vi "Array.vi"() -> (2 "Startlinie true":bool, 3 "array":bool[](array[boolean]))   [LabVIEW 2016]
doc: "VI berrechnet Abweichung des Linearray zur Mittellinie\n05.04.17_Tloe"
uses:
  <vilib>/myRIO/Instrument Drivers/Onboard IO/DIO/typedefs/DIO Reference.ctl
  <vilib>/myRIO/Common/Instrument Driver Framework/Utilities/typedefs/myRIO Generic Hardware Reference.ctl
  <vilib>/myRIO/Common/Instrument Driver Framework/Utilities/typedefs/Hardware Version Enum.ctl
  <vilib>/myRIO/Common/Instrument Driver Framework/Utilities/typedefs/myRIO v1.0 Reference.ctl
  <vilib>/myRIO/Common/Instrument Driver Framework/Utilities/typedefs/Generic FPGA Reference.ctl
  <vilib>/myRIO/Common/Instrument Driver Framework/myRIO v1.0/DIO/typedefs/DIO Channels List.ctl
  <vilib>/myRIO/Common/Instrument Driver Framework/myRIO v1.0/DIO/typedefs/DIO Channels Enum.ctl
  <vilib>/userdefined/High Color/nirio_resource_hc.ctl
  <vilib>/myRIO/Common/Instrument Driver Framework/Utilities/vis/Is FPGA Ref Available.vi
  <vilib>/myRIO/Common/Instrument Driver Framework/myRIO v1.0/DIO/vis/myRIO v1.1 Open DIO.vi
  <vilib>/myRIO/Instrument Drivers/Onboard IO/DIO/vis/Read.vi
  <vilib>/myRIO/Common/Instrument Driver Framework/Utilities/vis/Validate Channels.vi
  <vilib>/myRIO/Common/Instrument Driver Framework/myRIO v1.0/DIO/vis/myRIO v1.0 Reserve DIO.vi
  <vilib>/myRIO/Common/Instrument Driver Framework/myRIO v1.0/Resource Manager/vis/myRIO v1.0 Reserve Channel List.vi
  <vilib>/myRIO/Common/Instrument Driver Framework/myRIO v1.0/DIO/vis/myRIO v1.0 Build MUX Configuration DIO.vi
  <vilib>/myRIO/Common/Instrument Driver Framework/myRIO v1.0/Resource Manager/vis/myRIO v1.0 Reserve Channel.vi
  <vilib>/myRIO/Common/Instrument Driver Framework/myRIO v1.0/Resource Manager/vis/myRIO v1.0 Unreserve Channel.vi
  <vilib>/myRIO/Common/Instrument Driver Framework/myRIO v1.0/Resource Manager/vis/myRIO v1.0 Create Configuration List.vi
  <vilib>/myRIO/Common/Instrument Driver Framework/myRIO v1.0/Resource Manager/vis/myRIO v1.0 Build Mutex Name.vi
  <vilib>/Utility/VariantDataType/GetNumericInfo.vi
  <vilib>/Utility/error.llb/Error Cluster From Error Code.vi
  <vilib>/myRIO/Common/Instrument Driver Framework/myRIO v1.0/myRIO v1.1 Open.vi
  <vilib>/myRIO/Common/Instrument Driver Framework/Utilities/vis/IO Manager.vi
  <vilib>/myRIO/Common/Instrument Driver Framework/Utilities/vis/Configuration Manager.vi
  <vilib>/myRIO/Common/Instrument Driver Framework/myRIO v1.0/Resource Manager/vis/myRIO v1.0 Configure IO.vi
  <vilib>/myRIO/Common/Instrument Driver Framework/myRIO v1.0/myRIO v1.0 Close.vi
  <vilib>/myRIO/Common/Instrument Driver Framework/myRIO v1.0/DIO/vis/myRIO v1.0 Read DIO.vi
  <vilib>/myRIO/Express VI/Onboard IO/DI/DI Express VI.xnode
  <vilib>/myRIO/Instrument Drivers/Onboard IO/DIO/vis/myRIO DIO Open.xnode
  <vilib>/myRIO/Instrument Drivers/Onboard IO/DIO/DIO.lvlib
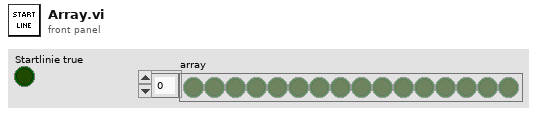
[diagram p1: front panel]
types:
  T1 = cluster{"A/DIO0 (Pin 11)":bool, "A/DIO1 (Pin 13)":bool, "A/DIO2 (Pin 15)":bool, "A/DIO3 (Pin 17)":bool, "A/DIO4 (Pin 19)":bool, "A/DIO5 (Pin 21)":bool, "A/DIO6 (Pin 23)":bool, "A/DIO7 (Pin 25)":bool, "B/DIO7 (Pin 25)":bool, "B/DIO6 (Pin 23)":bool, "B/DIO5 (Pin 21)":bool, "B/DIO3 (Pin 17)":bool, "B/DIO4 (Pin 19)":bool, "B/DIO2 (Pin 15)":bool, "B/DIO1 (Pin 13)":bool, "B/DIO12 (Pin 22)":bool}
  T2 = cluster{"A/DIO0 (Pin 11)":i16, "A/DIO1 (Pin 13)":i16, "A/DIO2 (Pin 15)":i16, "A/DIO3 (Pin 17)":i16, "A/DIO4 (Pin 19)":i16, "A/DIO5 (Pin 21)":i16, "A/DIO6 (Pin 23)":i16, "A/DIO7 (Pin 25)":i16, "B/DIO7 (Pin 25)":i16, "B/DIO6 (Pin 23)":i16, "B/DIO5 (Pin 21)":i16, "B/DIO3 (Pin 17)":i16, "B/DIO4 (Pin 19)":i16, "B/DIO2 (Pin 15)":i16, "B/DIO1 (Pin 13)":i16, "B/DIO12 (Pin 22)":i16}
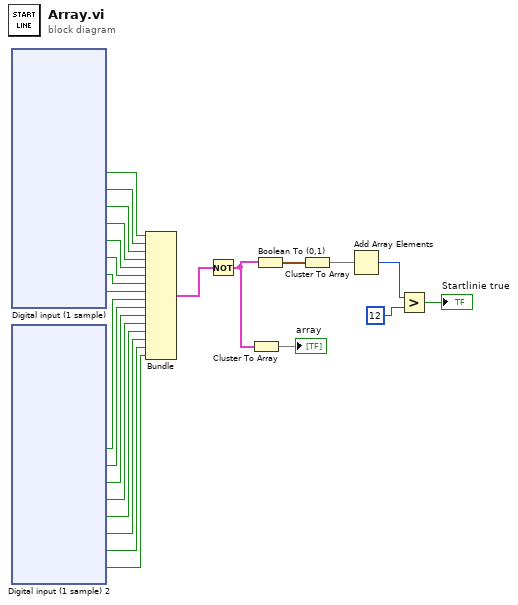
[diagram p0: block diagram]
diagram:
  n1 = xnode "Digital input (1 sample)"() -> ("A/DIO0 (Pin 11)"=w15:bool, "A/DIO1 (Pin 13)"=w16:bool, "A/DIO2 (Pin 15)"=w17:bool, "A/DIO3 (Pin 17)"=w18:bool, "A/DIO4 (Pin 19)"=w19:bool, "A/DIO5 (Pin 21)"=w20:bool, "A/DIO6 (Pin 23)"=w21:bool, "A/DIO7 (Pin 25)"=w22:bool)  [unwired: 1 in, 1 out]
  n2 = xnode "Digital input (1 sample) 2"() -> ("B/DIO7 (Pin 25)"=w11:bool, "B/DIO6 (Pin 23)"=w10:bool, "B/DIO5 (Pin 21)"=w9:bool, "B/DIO3 (Pin 17)"=w8:bool, "B/DIO4 (Pin 19)"=w7:bool, "B/DIO2 (Pin 15)"=w6:bool, "B/DIO1 (Pin 13)"=w5:bool, "B/DIO12 (Pin 22)"=w4:bool)  [unwired: 1 in, 1 out]
  n3 = Bundle("A/DIO0 (Pin 11)"=w15, "A/DIO1 (Pin 13)"=w16, "A/DIO2 (Pin 15)"=w17, "A/DIO3 (Pin 17)"=w18, "A/DIO4 (Pin 19)"=w19, "A/DIO5 (Pin 21)"=w20, "A/DIO6 (Pin 23)"=w21, "A/DIO7 (Pin 25)"=w22, "B/DIO7 (Pin 25)"=w11, "B/DIO6 (Pin 23)"=w10, "B/DIO5 (Pin 21)"=w9, "B/DIO3 (Pin 17)"=w8, "B/DIO4 (Pin 19)"=w7, "B/DIO2 (Pin 15)"=w6, "B/DIO1 (Pin 13)"=w5, "B/DIO12 (Pin 22)"=w4) -> (w14:T1)  [unwired: 1 in]
  n4 = Not(x=w14) -> (.not. x?=w2:T1)
  n5 = Cluster To Array(cluster=w2) -> (array=→"array":bool[])
  n6 = Boolean To (0,1)(Boolean=w2) -> (0, 1=w23:T2)
  n7 = Cluster To Array(cluster=w23) -> (array=w13:i16[])
  n8 = Add Array Elements(numeric array=w13) -> (sum=w12:i16)
  n9 = Greater?(x=w12, y=i16 12) -> (0:→"Startlinie true":bool)
